vi "POV.vi"() -> ()   [LabVIEW 2016]
panel:
  out "POV":dbl
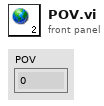
[diagram p1: front panel]
diagram:
